vi "lr1v15,no v3.vi"() -> ()   [LabVIEW 2012]
uses:
  <vilib>/express/express arith-compare/Formula/XNode/ExpressFormulaBlockNode.xnode
panel:
  out "ôóíò ñèëà íà ä^2":dbl(slide) scale=0.0..2.0
  out "ìì. Ðò. ñò":dbl(slide) scale=0.0..100000.0
  in  "Pa":dbl(slide) scale=0.0..1000.0
  in  "Boolean":bool
  # "Ñòîëá"
  # "Ôóíò"
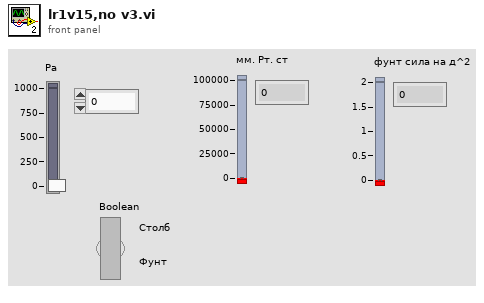
[diagram p1: front panel]
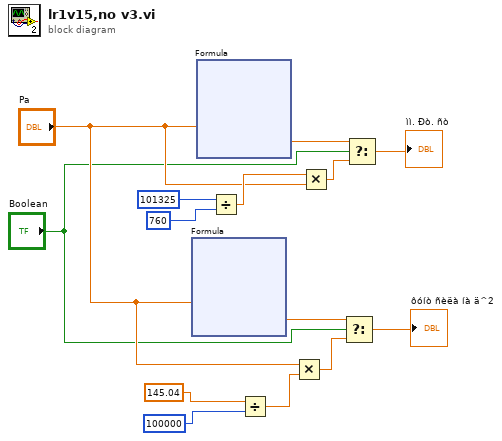
[diagram p0: block diagram]
diagram:
  n1 = xnode "Formula"("Pa"="Pa") -> ("Result"=w4:dbl)  [unwired: 1 in, 1 out]
  n2 = xnode "Formula"("Pa"="Pa") -> ("Result"=w10:dbl)  [unwired: 1 in, 1 out]
  n3 = Divide(x=101325, y=760) -> (x/y=w12:dbl)
  n4 = Divide(x=145.04, y=100000) -> (x/y=w7:dbl)
  n5 = Multiply(x="Pa", y=w7) -> (x*y=w5:dbl)
  n6 = Multiply(x=w12, y="Pa") -> (x*y=w11:dbl)
  n7 = Select(t=w4, s="Boolean", f=w5) -> (s? t:f=→"ôóíò ñèëà íà ä^2":dbl)
  n8 = Select(t=w10, s="Boolean", f=w11) -> (s? t:f=→"ìì. Ðò. ñò":dbl)
